vi "test_Add Command_Empty Command Format Error.vi"(8 "error in (no error)":errorcluster, 11 "TestCase in":refnum<class "Instrument Addon Scripting API Messages Unit Tests.lvclass">) -> (0 "error out":errorcluster, 3 "TestCase out":refnum<class "Instrument Addon Scripting API Messages Unit Tests.lvclass">)   [LabVIEW 2018, in "Instrument Addon Scripting API Messages Unit Tests.lvclass"]
uses:
  Instrument Addon Scripting API Messages Unit Tests.lvclass
  APIs/Scripting API/TypeDefs/Command Settings.ctl
  <vilib>/NI Veristand/Custom Device API/Custom Device Item Ref.ctl
  APIs/Scripting API/TypeDefs/Padding.ctl
  Addon/Addon Shared/SubVIs/Constants.vi
  <vilib>/NI/NI VeriStand Advanced SysDef API/_SubVIs/SysDef.Search.GUID.vi
  <vilib>/addons/_JKI Toolkits/VI Tester/TestCase.llb/TestCase.lvclass
  Instrument Addon Scripting API Test Assets/Instrument Addon Scripting API Test Assets.lvclass
  APIs/Scripting API/Instrument Addon Scripting API.lvlib
  <vilib>/NI/NI VeriStand Advanced SysDef API/SysDef API/Advanced System Definition.lvlib
  Addon/Addon Shared/Instrument Addon Shared.lvlib
  <vilib>/NI VeriStand/Custom Device API/Custom Device API.lvlib
  C:/Program Files (x86)/National Instruments/LabVIEW 2018/vi.lib/addons/_JKI Toolkits/VI Tester/TestCase.llb/TestCase.lvclass
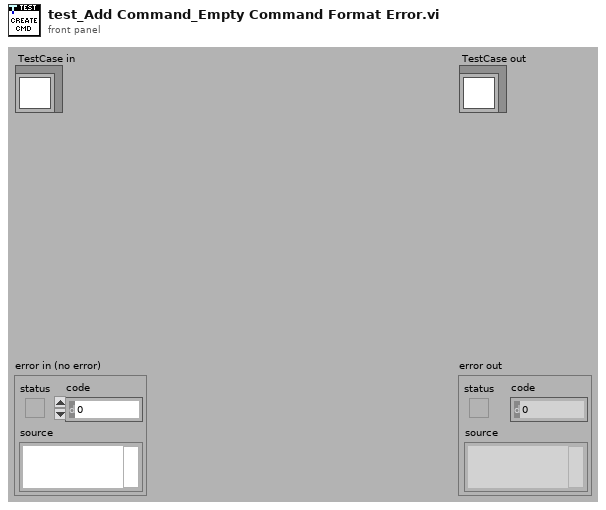
[diagram p1: front panel]
types:
  T1 = typedef "Custom Device API.lvlib/Custom Device Item Ref.ctl" = u64
  T2 = cluster{"Variable Name":string, "Channel Ref in":T1}[]
  T3 = typedef "Instrument Addon Scripting API.lvlib/Command Settings.ctl" = cluster{"Command Format":string, "Linked Channels":cluster{"Variable Name":string, "Channel Ref in":T1}[], "Use Padding?":bool, "Padding":T4}
  T4 = typedef "Instrument Addon Scripting API.lvlib/Padding.ctl" = cluster{"Pad Value":u8, "Length":u32}
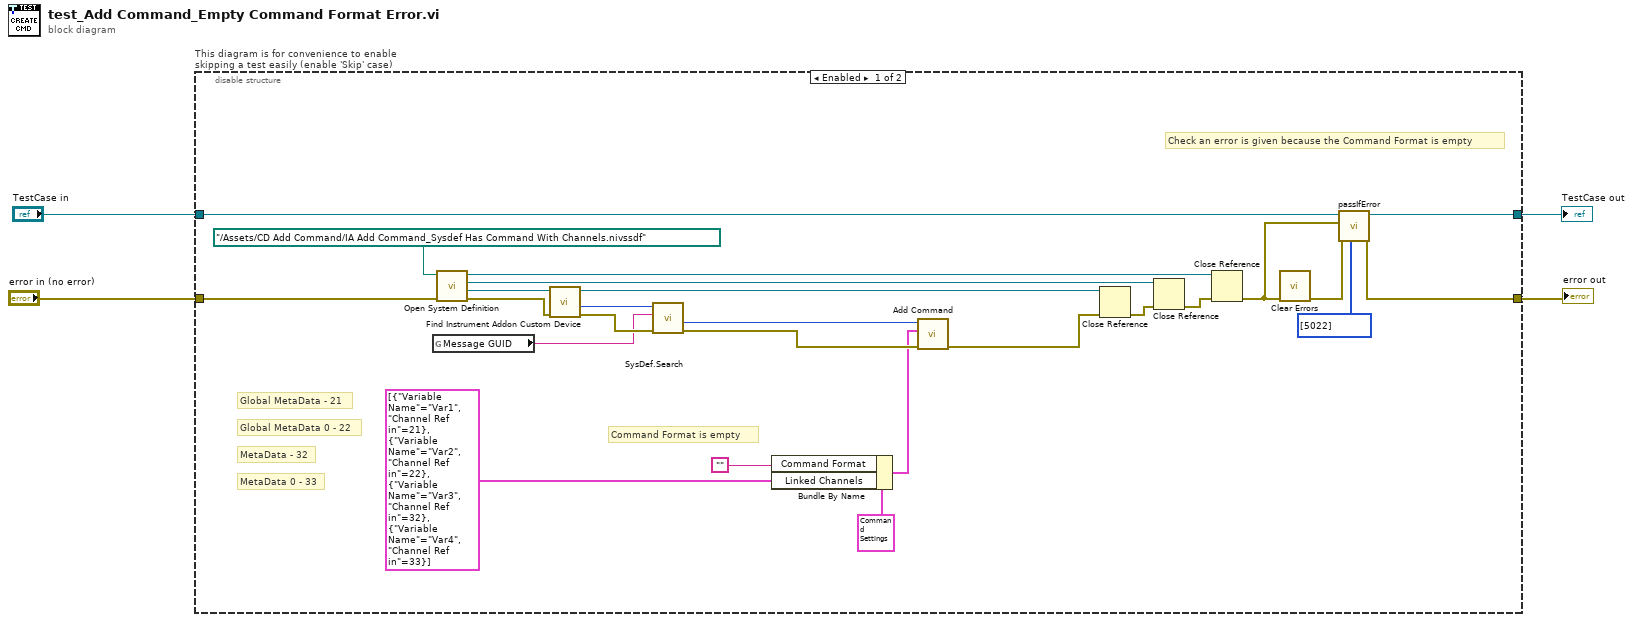
[diagram p0: block diagram]
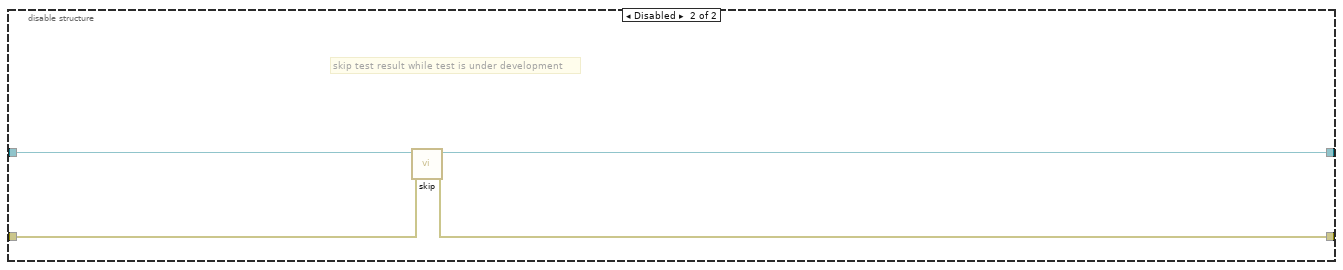
[diagram p2: hidden frame]
diagram:
  n1 = disable-structure "This diagram is for convenience to enable skipping a test easily (enable 'Skip' case)" shown="Enabled" {
    disable-tunnel: "TestCase in" -> [w26 w33]
    disable-tunnel: [w23 w31] -> w1
    disable-tunnel: [w24 w32] -> w3
    disable-tunnel: "error in (no error)" -> [w28 w30]
    frame Enabled {
      # "Command Format is empty"
      # "Check an error is given because the Command Format is empty"
      # "MetaData 0 - 33"
      # "MetaData - 32"
      # "Global MetaData 0 - 22"
      # "Global MetaData - 21"
      n2 = global read "Constants.vi" "Message GUID"() -> (w16:string)
      n3 = call "Open System Definition.vi"("error in (no error)"=w28, "System Definition File"=path "../Assets/CD Add Command/IA Add Command_Sysdef Has Command With Channels.nivssdf" ("SDF file")) -> ("error out"=w18:errorcluster, "Target Refnum"=w19:refnum<k24>, "Root Refnum"=w27:refnum<k24>, "System Definition Refnum"=w21:refnum<k24>)  [unwired: 6 in]
      n4 = call "Find Instrument Addon Custom Device.vi"("error in"=w18, "target in"=w19) -> ("error out"=w17:errorcluster, "NodeID"=w9:u64, "target out"=w10:refnum<k24>)  [unwired: 7 in]
      n5 = call-poly <vilib>:"SysDef.Search.vi"("error in (no error)"=w17, "GUID"=w16, "nodeID"=w9) -> ("error out"=w14:errorcluster, "Value out"=w15:u64)  [unwired: 5 in, 2 out]
      n6 = Bundle By Name(cluster=T3 {"Command Format"="[Var1]+[Var2]", "Linked Channels"=[{"Variable Name"="Var1", "Channel Ref in"=32}, {"Variable Name"="Var2", "Channel Ref in"=33}], "Use Padding?"=FALSE, "Padding"={"Pad Value"=0, "Length"=0}} ("Settings"), "Command Format"="", "Linked Channels"=T2 [{"Variable Name"="Var1", "Channel Ref in"=21}, {"Variable Name"="Var2", "Channel Ref in"=22}, {"Variable Name"="Var3", "Channel Ref in"=32}, {"Variable Name"="Var4", "Channel Ref in"=33}]) -> (w12:T3)
      n7 = call "Add Command.vi"("Error In"=w14, "Settings"=w12, "Message Refnum In"=w15) -> ("Error Out"=w20:errorcluster)  [unwired: 6 in, 2 out]
      n8 = Close Reference(reference=w10, error in (no error)=w20) -> (error out=w22:errorcluster)
      n9 = Close Reference(reference=w27, error in (no error)=w22) -> (error out=w25:errorcluster)
      n10 = Close Reference(reference=w21, error in (no error)=w25) -> (error out=w6:errorcluster)
      n11 = call <vilib>:"Clear Errors.vi"("error in (no error)"=w6) -> ("error out"=w7:errorcluster)  [unwired: 5 in, 1 out]
      n12 = call-dynamic "passIfError.vi"("passing error codes (default = any error code)"=i32[] [5022], "error in (no error)"=w7, "error"=w6, "TestCase in"=w26) -> ("error out"=w24:errorcluster, "TestCase out"=w23:refnum<class "Instrument Addon Scripting API Messages Unit Tests.lvclass">)  [unwired: 6 in]
    }
    frame Disabled {
      # "skip test result while test is under development"
      n13 = call <vilib>:"skip.vi"("error in (no error)"=w30, "TestCase in"=w33) -> ("error out"=w32:errorcluster, "TestCase out"=w31:refnum<class "Instrument Addon Scripting API Messages Unit Tests.lvclass">)  [unwired: 8 in]
    }
  }
  "error out" <- w3
  "TestCase out" <- w1
